vi "reg-log-general.vi"(6 "Operation(Read)":T3, 8 "error in":errorcluster, 10 "filter by proc name":string, 11 "Reports to Collect":T4 {"clk" format="%#.3f"}) -> (0 "error out":errorcluster, 2 "compact report":T1[](array[typedef]) {"clk" format="%#.1f"}, 3 "Collected Reports":T4[](array[typedef]) {"clk" format="%#.3f"})   [LabVIEW 2024]
uses:
  controls/typeEngineLogCluster.ctl
  controls/type.StepFunction.ctl
  controls/enum.report-filter.ctl
  controls/UiCompactReport.ctl
panel:
  out "size(s)":i32
  in  "Rows":i32=100
  # "stepIndex>=0 then filter by step index\nstepIndex==-1 then do not filter"
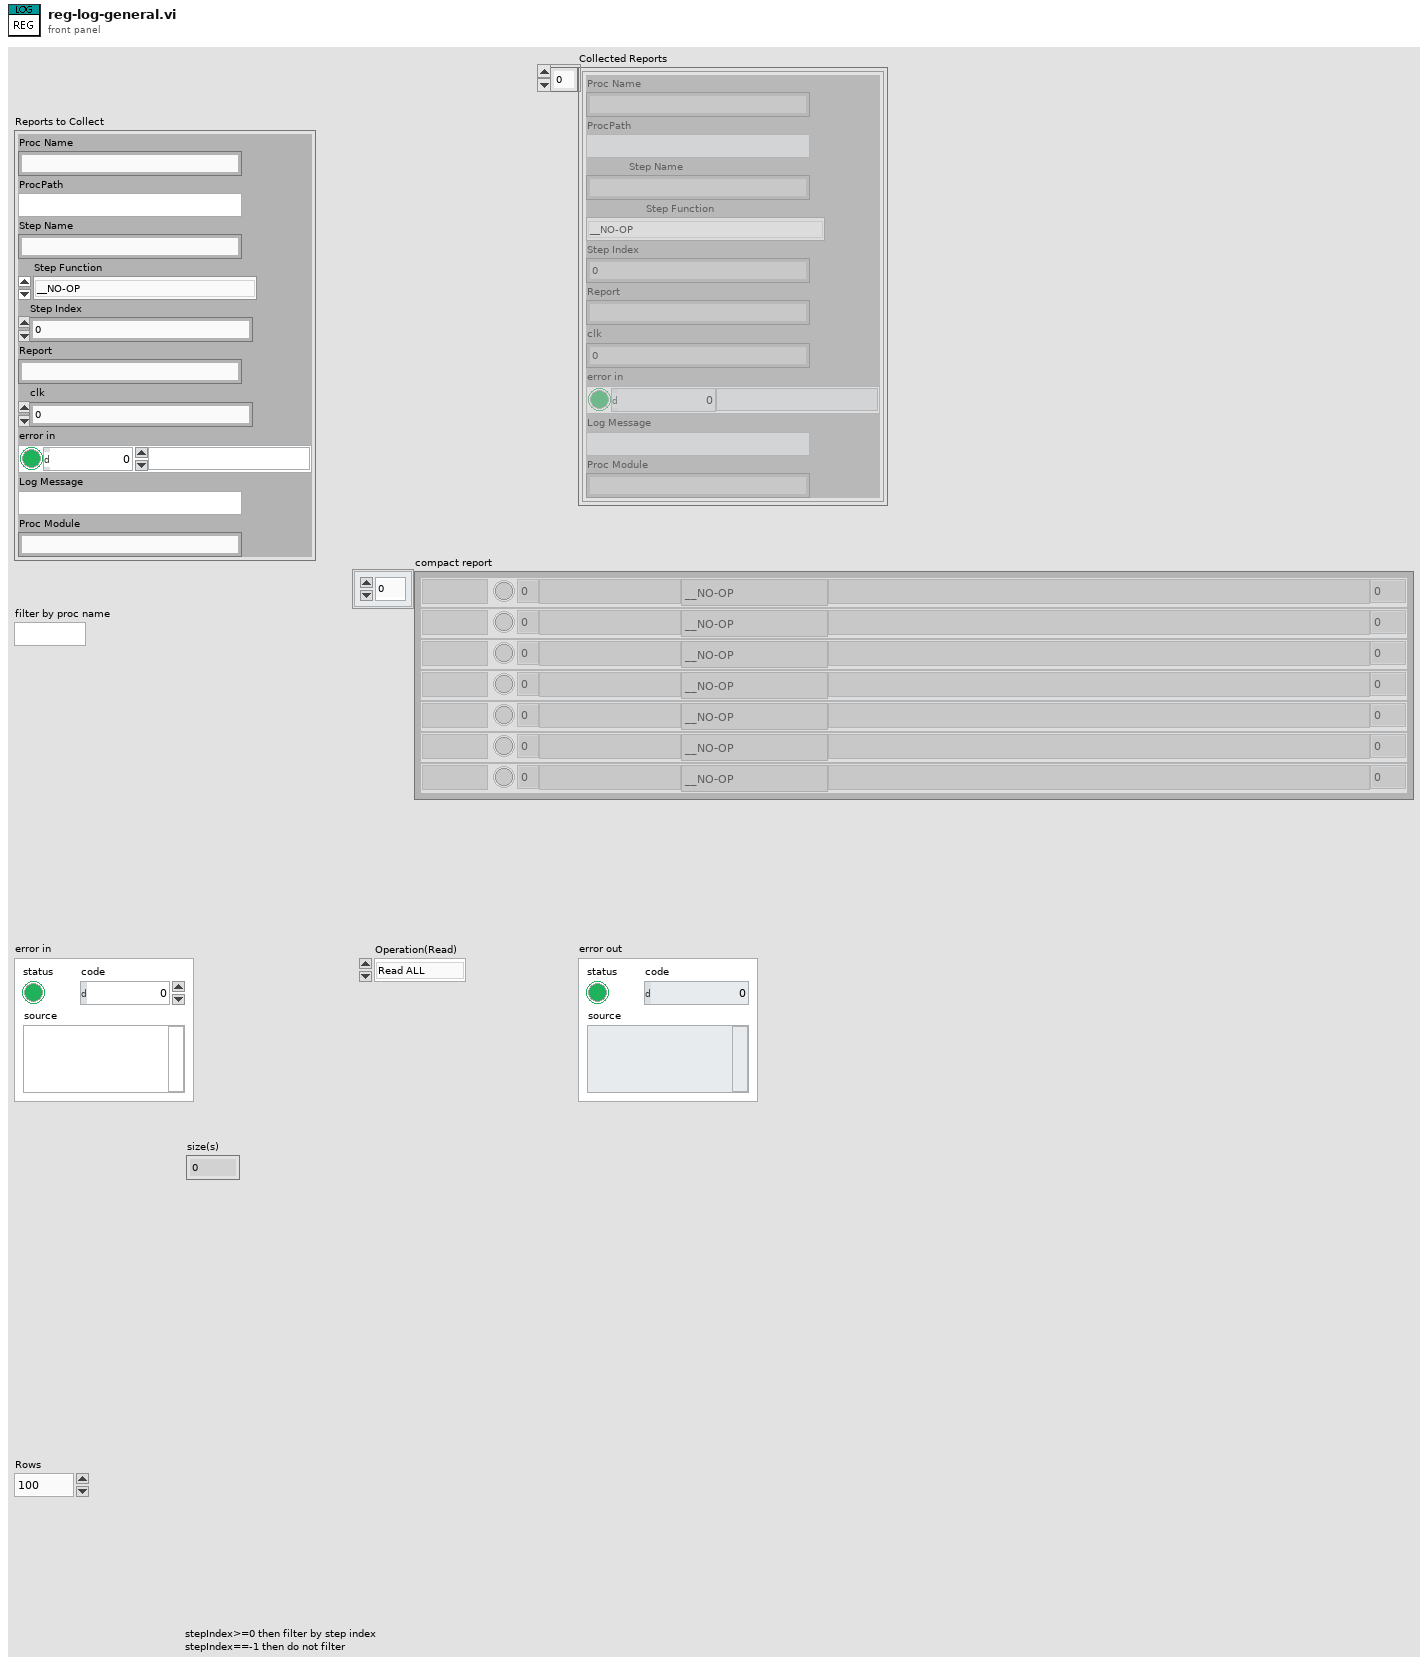
[diagram p1: front panel]
types:
  T1 = typedef "UiCompactReport.ctl" = cluster{"ErrorFlag":bool, "idx":i32, "Step Name":string, "Step Function":T2, "Report":string, "clk":dbl, "Proc":string}
  T2 = typedef "type.StepFunction.ctl" = enum16{"__NO-OP", "_DELAY_LOAD", "_DELAY_COMPARE", "_JUMP", "_COMPLETE", "_COMPARE", "_LOG_MESSAGE", "_LOG_LAST_REPORT", "_SCHEDULE", "_SCHED_DAILY", "CLK_COMPARE", "PROC_START", "PROC_STOP", "PROC_LOAD", "PROC_COMPLETION_CHECK", "PROC_COMPLETION_LOAD", "_IO_READ", "_IO_READ_MANY", "_IO_WRITE", "_IO_WRITE_BY_REG", "_IO_GET_OUTPUT", "_OCS_CHECK", "_OCS_RECORD", "_GET_RH", "_GET_ACC_UV", "_GET_WD", "_GET_WS", "_REC_DELETE", "_REC_MOVE", "_REC_COPY", "_IRR_CHECK", "UNIT_CHECK", "UNIT_SAMPLE", "UNIT_DOSE"}
  T3 = typedef "enum.report-filter.ctl" = enum16{"Read ALL", "Read Errors", "Collect", "ClearAll"}
  T4 = typedef "typeEngineLogCluster.ctl" = cluster{"Proc Name":string, "ProcPath":string, "Step Name":string, "Step Function":T2, "Step Index":i32, "Report":string, "clk":dbl, "error in":errorcluster, "Log Message":string, "Proc Module":string}
  T5 = cluster{"Proc Name":bool, "ProcPath":bool, "Step Name":bool, "Step Function":bool, "Step Index":bool, "Report":bool, "clk":bool, "error in":cluster{"status":bool, "code":bool, "source":bool}, "Log Message":bool, "Proc Module":bool}
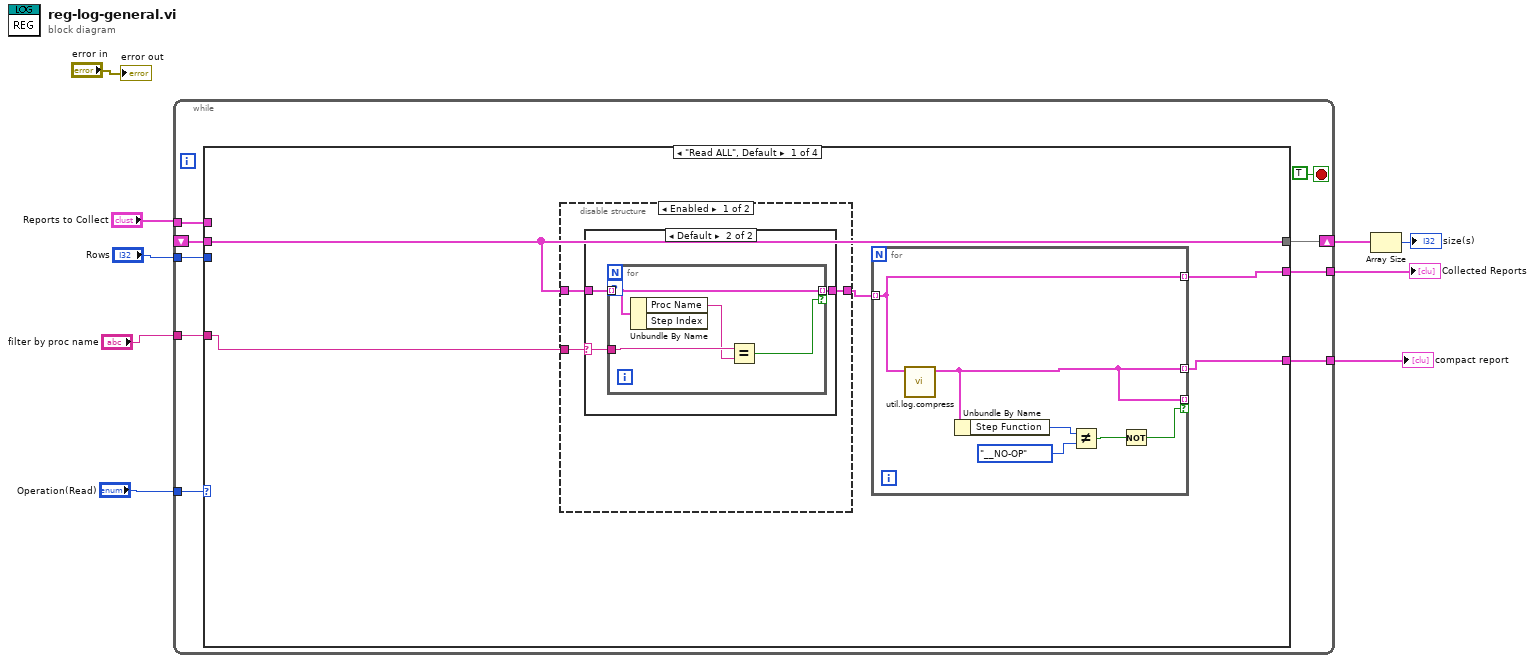
[diagram p0: block diagram]
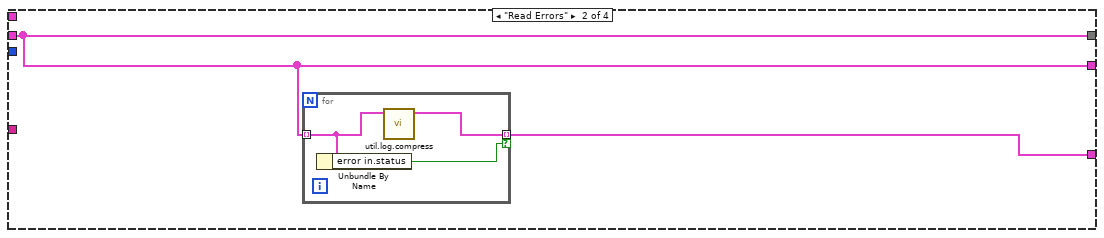
[diagram p4: hidden frame]
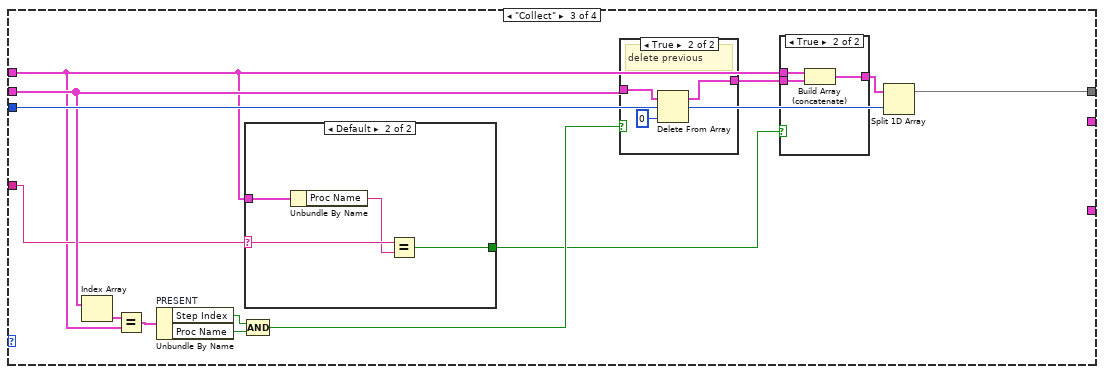
[diagram p5: hidden frame]
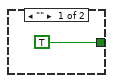
[diagram p7: hidden frame]
diagram:
  n1 = while {
    shift-right: [w16] -> w6
    shift-left: _ -> [w14]
    tunnel: "Reports to Collect" -> [w18]
    tunnel: "Rows" -> [w15]
    tunnel: "Operation(Read)" -> [w13]
    tunnel: [w12] -> w4
    tunnel: [w11] -> w3
    tunnel: "filter by proc name" -> [w10]
    stop <- TRUE stop-if-true
    n2 = case shown="\"Read ALL\", Default" w13 {
      tunnel: w18 -> [_ _ w48 _]
      tunnel: [w23 w43 w59 _] -> w16
      tunnel: w15 -> [_ _ w58 _]
      tunnel: w14 -> [w23 w43 w57 _]
      tunnel: [w22 w43 _ _] -> w12
      tunnel: [w19 w42 _ _] -> w11
      tunnel: w10 -> [w21 _ w49 _]
      frame "Read ALL", Default {
        n3 = disable-structure shown="Enabled" {
          disable-tunnel: w23 -> [w26 w35]
          disable-tunnel: w21 -> [w24 _]
          disable-tunnel: [w25 w35] -> w20
          frame Enabled {
            n4 = case shown="Default" w24 {
              selector: w24 -> [_ w28]
              tunnel: w26 -> [w27 w30]
              tunnel: [w27 w29] -> w25
              frame "" {
              }
              frame Default {
                n5 = for {
                  tunnel: w30 -> [w31] mode=indexing
                  tunnel: w28 -> [w34]
                  tunnel: [w31] -> w29 mode=indexing if=w33
                  workers-P: _ -> [_]
                  n6 = Unbundle By Name(w31) -> ("Proc Name"=w32:string)  [unwired: 1 out]
                  n7 = Equal?(x=w34, y=w32) -> (x = y?=w33:bool)
                }
              }
            }
          }
          frame Disabled {
          }
        }
        n8 = for {
          tunnel: w20 -> [w41] mode=indexing
          tunnel: [w41] -> w22 mode=indexing
          tunnel: [w38] -> w19 mode=indexing
          tunnel: [w38] -> _ mode=indexing if=w36
          n9 = call "util.log.compress.vi"("Log Cluster in"=w41) -> ("Compact Report"=w38:T1)  [unwired: 9 in, 1 out]
          n10 = Unbundle By Name(w38) -> ("Step Function"=w39:T2)
          n11 = Not Equal?(x=w39, y=type.StepFunction."__NO-OP" ("Step Function")) -> (x != y?=w37:bool)
          n12 = Not(x=w37) -> (.not. x?=w36:bool)
        }
      }
      frame "Read Errors" {
        n13 = for {
          tunnel: w43 -> [w45] mode=indexing
          tunnel: [w46] -> w42 mode=indexing if=w44
          n14 = Unbundle By Name(w45) -> ("error in.status"=w44:bool)
          n15 = call "util.log.compress.vi"("Log Cluster in"=w45) -> ("Compact Report"=w46:T1)  [unwired: 9 in, 1 out]
        }
      }
      frame "Collect" {
        n16 = Index Array(array=w57) -> (element=w50:T4)  [unwired: 1 in]
        n17 = Equal?(x=w50, y=w48) -> (x = y?=w53:T5)
        n18 = Unbundle By Name "PRESENT"(w53) -> ("Step Index"=w51:bool, "Proc Name"=w52:bool)
        n19 = case shown="Default" w49 {
          selector: w49 -> [_ w67]
          tunnel: w48 -> [_ w68]
          tunnel: [TRUE ("Boolean") w65] -> w47
          frame "" {
          }
          frame Default {
            n20 = Unbundle By Name(w68) -> ("Proc Name"=w66:string)
            n21 = Equal?(x=w67, y=w66) -> (x = y?=w65:bool)
          }
        }
        n22 = Compound Arithmetic op=AND(w51, w52) -> (w54:bool)
        n23 = case shown="True" w54 {
          tunnel: w57 -> [w69 w72]
          tunnel: [w69 w71] -> w56
          frame False {
          }
          frame True {
            # "delete previous"
            n24 = Delete From Array(array=w72, index=0) -> (array with subset deleted=w71:T4[])  [unwired: 1 in, 1 out]
          }
        }
        n25 = case shown="True" w47 {
          tunnel: w56 -> [w60 w63]
          tunnel: [w60 w62] -> w55
          tunnel: w48 -> [_ w61]
          frame False {
          }
          frame True {
            n26 = Build Array (concatenate)(w61, w63) -> (w62:T4[])
          }
        }
        n27 = Split 1D Array(array=w55, index=w58) -> (first subarray=w59:T4[])  [unwired: 1 out]
      }
      frame "ClearAll" {
      }
    }
  }
  "Collected Reports" <- w4
  "compact report" <- w3
  n28 = Array Size(array=w6) -> (size(s)=→"size(s)":i32)
  "error out" <- "error in"
